vi "get_terminals.vi"(0 "ClockDL100201DAQmx in":refnum<class "ClockDL100201DAQmx.lvclass">, 11 "error in (no error)":errorcluster) -> (4 "ClockDL100201DAQmx out":refnum<class "ClockDL100201DAQmx.lvclass">, 6 "output terminal":tag, 8 "trigger source":tag, 10 "period counter":tag, 15 "error out":errorcluster)   [LabVIEW 2010, in "ClockDL100201DAQmx.lvclass"]
uses:
  ClockDL100201DAQmx.lvclass
  ClockDL100201DAQmx.lvclass/ClockDL100201DAQmx.ctl
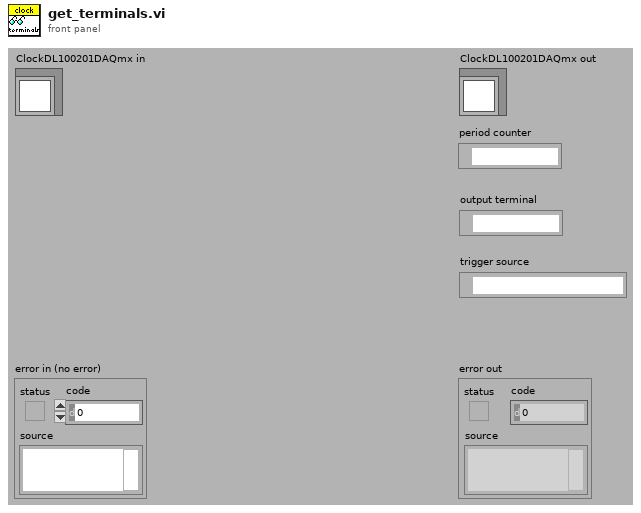
[diagram p1: front panel]
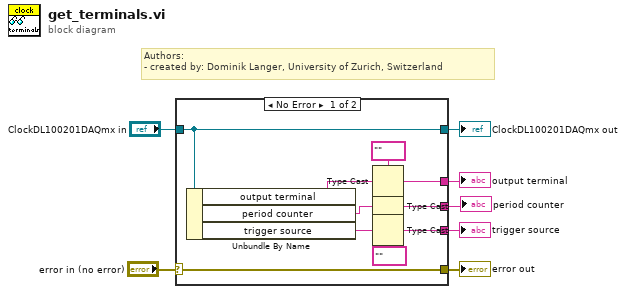
[diagram p0: block diagram]
diagram:
  # "Authors: \n- created by: Dominik Langer, University of Zurich, Switzerland"
  n1 = case shown="No Error" "error in (no error)" {
    selector: "error in (no error)" -> [w17 w19]
    tunnel: [w17 w19] -> w6
    tunnel: [w15 w18] -> w4
    tunnel: "ClockDL100201DAQmx in" -> [w15 w18]
    tunnel: [w14 _] -> w3
    tunnel: [w13 _] -> w2
    tunnel: [w10 _] -> w1
    frame No Error {
      w9 = tag "" ("counter")
      n2 = Unbundle By Name(w15) -> ("output terminal"=w16:string, "period counter"=w11:string, "trigger source"=w12:string)
      n3 = Type Cast(type=w9, x=w16) -> (*(type *) &x=w14:tag)
      n4 = Type Cast(type=w9, x=w11) -> (*(type *) &x=w10:tag)
      n5 = Type Cast(type=tag "" ("source"), x=w12) -> (*(type *) &x=w13:tag)
    }
    frame Error {
    }
  }
  "error out" <- w6
  "ClockDL100201DAQmx out" <- w4
  "output terminal" <- w3
  "trigger source" <- w2
  "period counter" <- w1
